vi "lvBuildAllTargets.vi"() -> (0 "error out":errorcluster)   [LabVIEW 2016, in "lvcommonbuild.lvlib"]
uses:
  lvcommonbuild.lvlib
  <vilib>/Wiresmith Technology/LabVIEW CLI/CLI Class/CLI.lvclass
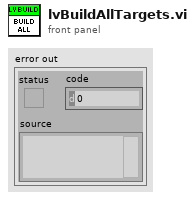
[diagram p1: front panel]
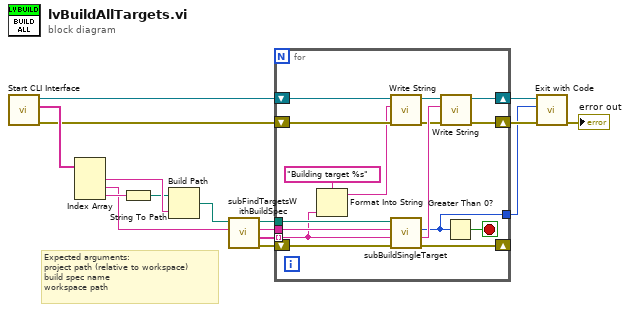
[diagram p0: block diagram]
diagram:
  # "Expected arguments:\nproject path (relative to workspace)\nbuild spec name\nworkspace path"
  n1 = call <vilib>:"Start CLI Interface.vi"() -> ("error out"=w3:errorcluster, "Custom Parameters"=w16:string[], "CLI out"=w5:refnum<class "CLI.lvclass">)  [unwired: 9 in]
  n2 = Index Array(array=w16) -> (element #1=w14:string, element #2=w10:string, element #3=w12:string)  [unwired: 3 in]
  n3 = String To Path(string=w12) -> (path=w13:path)
  n4 = Build Path(base path=w13, name or relative path=w14) -> (appended path=w11:path)
  n5 = call "subFindTargetsWithBuildSpec.vi"("Build Spec Name"=w10, "Project"=w11) -> ("error out"=w9:errorcluster, "Targets with spec name"=w6:string[], "dup Build Spec Name"=w7:string, "dup Project"=w8:path)  [unwired: 6 in]
  n6 = for {
    tunnel: w8 -> [w31]
    tunnel: w7 -> [w30]
    tunnel: w6 -> [w19] mode=indexing
    shift-right: [w29] -> w4
    shift-left: w5 -> [w21]
    shift-right: [w27] -> _
    shift-left: w9 -> [w32]
    shift-right: [w26] -> w2
    shift-left: w3 -> [w23]
    tunnel: [w24] -> w1
    stop <- w25 stop-if-true
    n7 = Format Into String(format string="Building target %s", w19) -> (resulting string=w17:string)  [unwired: 2 in, 1 out]
    n8 = call <vilib>:"Write String.vi"("error in (no error)"=w23, "Text to Write"=w17, "CLI in"=w21) -> ("error out"=w22:errorcluster, "CLI out"=w20:refnum<class "CLI.lvclass">)  [unwired: 7 in]
    n9 = call "subBuildSingleTarget.vi"("error in (no error)"=w32, "Target"=w19, "Build Spec"=w30, "Project"=w31) -> ("error out"=w27:errorcluster, "Output Message"=w28:string, "Exit Code (0)"=w24:i32)  [unwired: 5 in]
    n10 = call <vilib>:"Write String.vi"("error in (no error)"=w22, "Text to Write"=w28, "CLI in"=w20) -> ("error out"=w26:errorcluster, "CLI out"=w29:refnum<class "CLI.lvclass">)  [unwired: 7 in]
    n11 = Greater Than 0?(x=w24) -> (x > 0?=w25:bool)
  }
  n12 = call <vilib>:"Exit with Code.vi"("error in (no error)"=w2, "Exit Code (0)"=w1, "CLI in"=w4) -> ("error out"=→"error out":errorcluster)  [unwired: 8 in]
